vi "ExSubCreateFileImageFastFileType.vi"(0 "Camera Handle":u32, 1 "Pulser Handle":u32, 2 "File and Display Name":string, 3 "error in (no error)":errorcluster) -> (5 "Handles Out":T1, 7 "error out":errorcluster)   [LabVIEW 2010]
panel:
  # "ExSubCreateFileMultImage.vi:\nThis is a SubVI that creates a file,  and image objects and returns the handles bundled in a cluster that includes a pulser and camera handle"
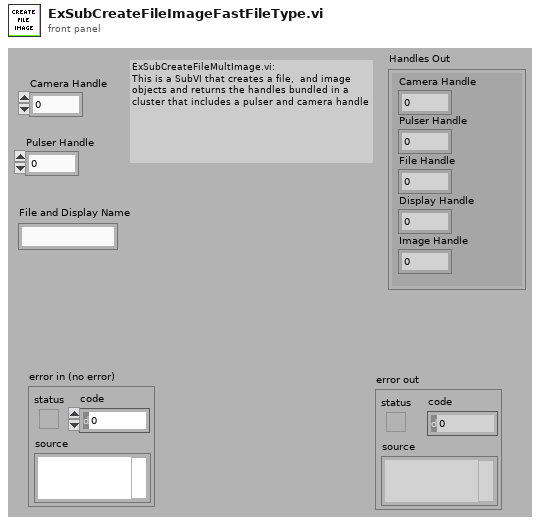
[diagram p1: front panel]
types:
  T1 = cluster{"Camera Handle":u32, "Pulser Handle":u32, "File Handle":u32, "Display Handle":u32, "Image Handle":u32}
  T2 = cluster{"Camera Handle":u32, "Pulser Handle":u32, "File Handle":u32, i32, "Image Handle":u32}
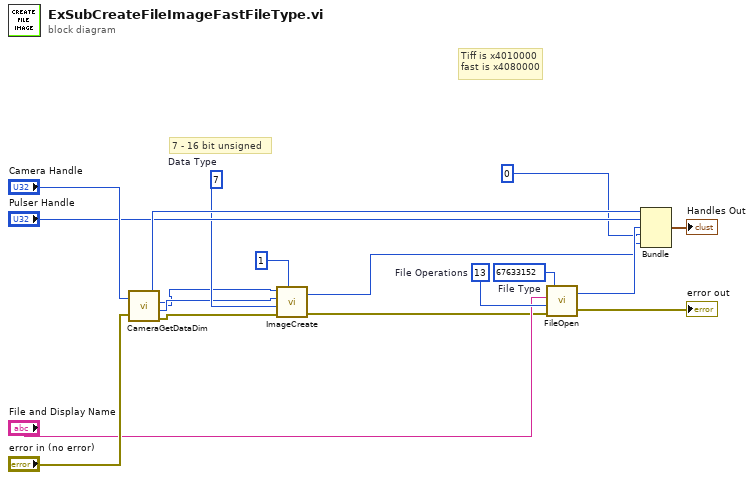
[diagram p0: block diagram]
diagram:
  w8 = u32 7  # Data Type
  w11 = 13  # File Operations
  w12 = 67633152  # File Type
  # "Tiff is x4010000\nfast is x4080000"
  # "7 - 16 bit unsigned"
  n1 = call <userlib>:"CameraGetDataDim.vi"("Camera Handle"="Camera Handle", "error in"="error in (no error)") -> ("Camera Handle"=w15:u32, "Xdim"=w4:u32, "Ydim"=w5:u32, "error out"=w7:errorcluster)
  n2 = call <userlib>:"ImageCreate.vi"("X dimension"=w4, "Y dimension"=w5, "Data Type"=w8, "error in"=w7, "Number Of Frames"=u32 1) -> ("Image Handle"=w2:u32, "error out"=w6:errorcluster)
  n3 = call <userlib>:"FileOpen.vi"("error in"=w6, "File Operations"=w11, "FileName"="File and Display Name", "File Type"=w12) -> ("error out"=→"error out":errorcluster, "File Handle"=w13:u32)
  n4 = Bundle("Camera Handle"=w15, "Pulser Handle"="Pulser Handle", "File Handle"=w13, 0, "Image Handle"=w2) -> (→"Handles Out":T2)  [unwired: 1 in]
